vi "Get Task List.vi"(8 "error in (no error)":errorcluster) -> (0 "error out":errorcluster, 3 "names of application windows":string[](array[string]))   [LabVIEW 2020, in "MacroAssert.lvlib" / "Winevent.lvlib"]
doc: "This VI lists Windows' currently running tasks."
uses:
  Winevent.lvlib
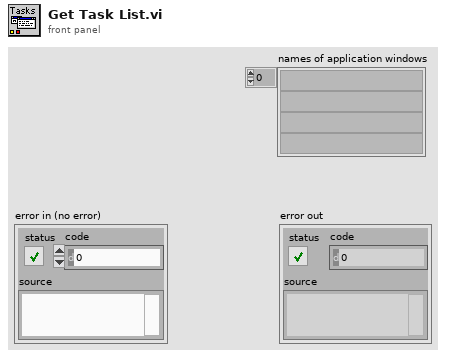
[diagram p1: front panel]
types:
  T1 = enum16{"Get Number of Tasks", "Get Window Info", "Get Window Names"}
  T2 = cluster{"number of windows":i32, "total names length":u32, "number of tasks found":i32, "window handles":u32[], "process ID":u32}
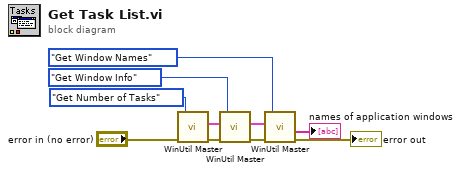
[diagram p0: block diagram]
diagram:
  n1 = call "WinUtil Master.vi"("error in (no error)"="error in (no error)", "function"=T1."Get Number of Tasks") -> ("error out"=w7:errorcluster, "window enumeration info out"=w6:T2)  [unwired: 1 in, 3 out]
  n2 = call "WinUtil Master.vi"("error in (no error)"=w7, "window enumeration info in"=w6, "function"=T1."Get Window Info") -> ("error out"=w5:errorcluster, "window enumeration info out"=w4:T2)  [unwired: 3 out]
  n3 = call "WinUtil Master.vi"("error in (no error)"=w5, "window enumeration info in"=w4, "function"=T1."Get Window Names") -> ("error out"=→"error out":errorcluster, "window names"=→"names of application windows":string[])  [unwired: 3 out]
